vi "IMAQdx Set Camera ROI.vi"(8 "error in (no error)":errorcluster, 10 "Desired ROI":T1, 11 "Session in":T2) -> (0 "error out":errorcluster, 2 "Actual ROI":T1, 3 "Session out":T2)   [LabVIEW 2020]
uses:
  <vilib>/userdefined/High Color/IMAQdx.ctl
  Rounding Mode.ctl
  <resource>/objmgr/imaqdx.rc
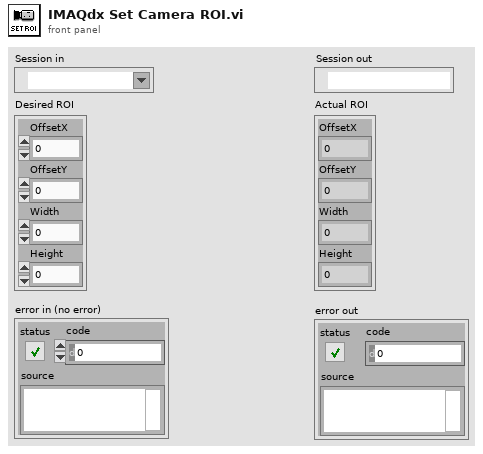
[diagram p1: front panel]
types:
  T1 = cluster{"OffsetX":i64, "OffsetY":i64, "Width":i64, "Height":i64}
  T2 = typedef "IMAQdx.ctl" = refnum<k21>
  T3 = typedef "Rounding Mode.ctl" = enum16{"Round to Nearest", "Round to Lowest", "Round to Highest"}
  T4 = cluster{"ValueI64":i64, "ValueI64":i64, "ValueI64":i64, "ValueI64":i64}
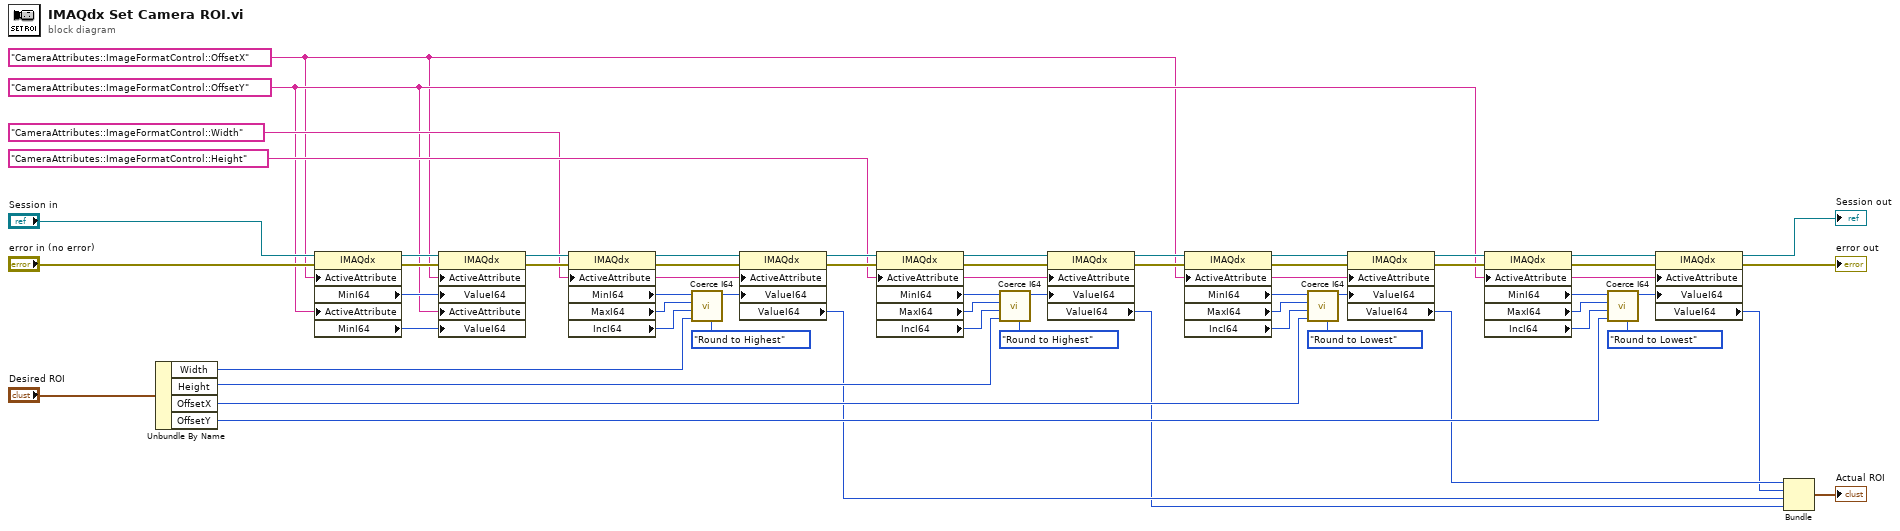
[diagram p0: block diagram]
diagram:
  w24 = "CameraAttributes::ImageFormatControl::Height" ("String")
  w17 = "CameraAttributes::ImageFormatControl::Width" ("String")
  w2 = "CameraAttributes::ImageFormatControl::OffsetY" ("String")
  w1 = "CameraAttributes::ImageFormatControl::OffsetX" ("String")
  n1 = Unbundle By Name("Desired ROI") -> ("Width"=w15:i64, "Height"=w14:i64, "OffsetX"=w13:i64, "OffsetY"=w12:i64)
  n2 = property class="IMAQdx"(reference="Session in", error in="error in (no error)", "ActiveAttribute"=w1, "ActiveAttribute"=w2) -> (reference out=w58:T2, error out=w57:errorcluster, "MinI64"=w3:i64, "MinI64"=w4:i64)
  n3 = property class="IMAQdx"(reference=w58, error in=w57, "ActiveAttribute"=w1, "ValueI64"=w3, "ActiveAttribute"=w2, "ValueI64"=w4) -> (reference out=w55:T2, error out=w56:errorcluster)
  n4 = property class="IMAQdx"(reference=w55, error in=w56, "ActiveAttribute"=w17) -> (reference out=w37:T2, error out=w36:errorcluster, "MinI64"=w33:i64, "MaxI64"=w34:i64, "IncI64"=w35:i64)
  n5 = call "Coerce I64.vi"("Rounding Mode (Round to Nearest))"=Rounding_Mode."Round to Highest", "Value"=w15, "Increment"=w35, "Maximum"=w34, "Minimum"=w33) -> ("Coerced Value"=w21:i64)  [unwired: 6 in]
  n6 = property class="IMAQdx"(reference=w37, error in=w36, "ActiveAttribute"=w17, "ValueI64"=w21) -> (reference out=w25:T2, error out=w26:errorcluster, "ValueI64"=w8:i64)
  n7 = property class="IMAQdx"(reference=w25, error in=w26, "ActiveAttribute"=w24) -> (reference out=w31:T2, error out=w30:errorcluster, "MinI64"=w27:i64, "MaxI64"=w28:i64, "IncI64"=w29:i64)
  n8 = call "Coerce I64.vi"("Rounding Mode (Round to Nearest))"=Rounding_Mode."Round to Highest", "Value"=w14, "Increment"=w29, "Maximum"=w28, "Minimum"=w27) -> ("Coerced Value"=w20:i64)  [unwired: 6 in]
  n9 = property class="IMAQdx"(reference=w31, error in=w30, "ActiveAttribute"=w24, "ValueI64"=w20) -> (reference out=w53:T2, error out=w54:errorcluster, "ValueI64"=w7:i64)
  n10 = property class="IMAQdx"(reference=w53, error in=w54, "ActiveAttribute"=w1) -> (reference out=w43:T2, error out=w42:errorcluster, "MinI64"=w39:i64, "MaxI64"=w40:i64, "IncI64"=w41:i64)
  n11 = call "Coerce I64.vi"("Rounding Mode (Round to Nearest))"=Rounding_Mode."Round to Lowest", "Value"=w13, "Increment"=w41, "Maximum"=w40, "Minimum"=w39) -> ("Coerced Value"=w23:i64)  [unwired: 6 in]
  n12 = property class="IMAQdx"(reference=w43, error in=w42, "ActiveAttribute"=w1, "ValueI64"=w23) -> (reference out=w50:T2, error out=w48:errorcluster, "ValueI64"=w10:i64)
  n13 = property class="IMAQdx"(reference=w50, error in=w48, "ActiveAttribute"=w2) -> (reference out=w52:T2, error out=w46:errorcluster, "MinI64"=w44:i64, "MaxI64"=w45:i64, "IncI64"=w49:i64)
  n14 = call "Coerce I64.vi"("Rounding Mode (Round to Nearest))"=Rounding_Mode."Round to Lowest", "Value"=w12, "Increment"=w49, "Maximum"=w45, "Minimum"=w44) -> ("Coerced Value"=w22:i64)  [unwired: 6 in]
  n15 = property class="IMAQdx"(reference=w52, error in=w46, "ActiveAttribute"=w2, "ValueI64"=w22) -> (reference out=→"Session out":T2, error out=→"error out":errorcluster, "ValueI64"=w9:i64)
  n16 = Bundle("ValueI64"=w10, "ValueI64"=w9, "ValueI64"=w8, "ValueI64"=w7) -> (→"Actual ROI":T4)  [unwired: 1 in]
